vi "read configuration file.vi"(11 "Template in":refnum<class "Template.lvclass">) -> (0 "error out":errorcluster, 2 "ActorConfiguration":T1={"GlobalConfiguration"={"DeviceFamily"="", "WriteData"=FALSE, "BufferSize_samples"=-1, "SyncDevice"=FALSE, "ExecuteInterruptRoutine"=FALSE, "InterruptRoutineTimeout_ms"=-1}, "DeviceConfiguration"={"DeviceSpecificName"="MIPI_Camera", "HardwareReference"="PXIe-Slot2", "UsedResources"=[{"ResourceLocation"="FrontFacing", "ResourceData"=variant(string "Use this Variant to store your specific resource data.\nThis will be read from and written to with the JSON parsing API.\nIn the child implementation you can use the acessors provided to convert from the specific cluster to your own device's implementation")}]}})   [LabVIEW 2020, in "Template.lvlib" / "Template.lvclass"]
doc: "Implements the configuration file reading.\nIf a file is not found, a new one is generated at .\\configs\\<actorName>_config.json"
uses:
  Template.lvclass
  typedefs/actor configuration.ctl
  typedefs/shared actor configuration.ctl
  typedefs/resource config/device configuration cluster.ctl
  typedefs/resource config/single resource cluster.ctl
  methods/read json file.vi/3c470e21-1639-4616-9875-34d8c0f16db8.vi
  methods/read json file.vi/465192f6-cf10-4ed9-8c5f-bfc9042509a2.vi
  <vilib>/Utility/file.llb/Application Directory.vi
  tools/return class name.vi
  <userlib>/_OpenG.lib/file/file.llb/Create Dir if Non-Existant__ogtk.vi
  <vilib>/JDP Science/JSONtext/JSON text to Variant.vi
  <vilib>/JDP Science/JSONtext/Variant to JSON Text.vi
  <vilib>/JDP Science/JSONtext/LVClass Serializer/JSONtext LVClass Serializer.lvclass
  Template.lvclass/Template.ctl
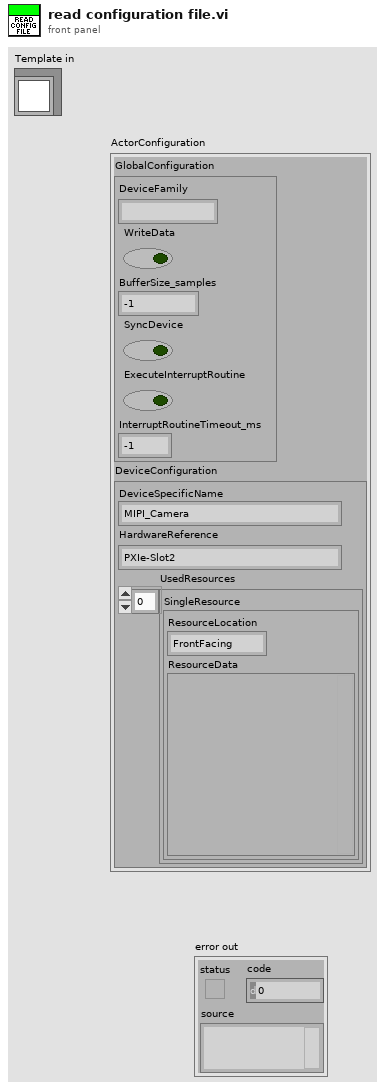
[diagram p1: front panel]
types:
  T1 = typedef "Template.lvlib/Template.lvclass/actor configuration.ctl" = cluster{"GlobalConfiguration":T2, "DeviceConfiguration":T3}
  T2 = typedef "Template.lvlib/Template.lvclass/shared actor configuration.ctl" = cluster{"DeviceFamily":string, "WriteData":bool, "BufferSize_samples":i32, "SyncDevice":bool, "ExecuteInterruptRoutine":bool, "InterruptRoutineTimeout_ms":i32}
  T3 = typedef "Template.lvlib/Template.lvclass/device configuration cluster.ctl" = cluster{"DeviceSpecificName":string, "HardwareReference":string, "UsedResources":T4[]}
  T4 = typedef "Template.lvlib/Template.lvclass/single resource cluster.ctl" = cluster{"ResourceLocation":string, "ResourceData":variant}
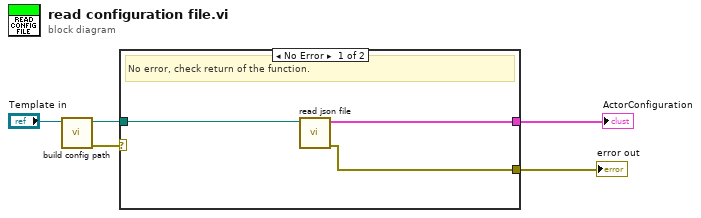
[diagram p0: block diagram]
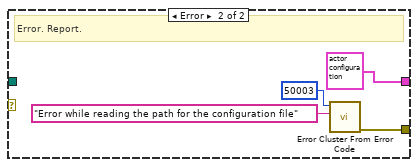
[diagram p2: hidden frame]
diagram:
  n1 = call "build config path.vi"("Template in"="Template in") -> ("error out"=w2:errorcluster, "Config Path"=w1:path)  [unwired: 9 in]
  n2 = case shown="No Error" w2 {
    tunnel: [w8 w12] -> w5
    tunnel: [w7 T1 {"GlobalConfiguration"={"DeviceFamily"="", "WriteData"=FALSE, "BufferSize_samples"=-1, "SyncDevice"=FALSE, "ExecuteInterruptRoutine"=FALSE, "InterruptRoutineTimeout_ms"=-1}, "DeviceConfiguration"={"DeviceSpecificName"="MIPI_Camera", "HardwareReference"="PXIe-Slot2", "UsedResources"=[{"ResourceLocation"="FrontFacing", "ResourceData"=variant(string "Use this Variant to store your specific resource data.\nThis will be read from and written to with the JSON parsing API.\nIn the child implementation you can use the acessors provided to convert from the specific cluster to your own device's implementation")}]}} ("Data out")] -> w3
    tunnel: w1 -> [w6 _]
    frame No Error {
      # "No error, check return of the function."
      n3 = call "read json file.vi"("File Path"=w6) -> ("error out"=w8:errorcluster, "Data out"=w7:T1)  [unwired: 9 in]
    }
    frame Error {
      # "Error. Report."
      n4 = call <vilib>:"Error Cluster From Error Code.vi"("error message (\"\")"="Error while reading the path for the configuration file" ("error message (\"\")"), "error code (0)"=50003) -> ("error out"=w12:errorcluster)  [unwired: 7 in]
    }
  }
  "error out" <- w5
  "ActorConfiguration" <- w3
